vi "Get Data.vi"(8 "Error In":errorcluster, 11 "Model in":refnum<class "Model.lvclass">) -> (0 "Error Out":errorcluster, 2 "Digital Data":u8[](array[numeric]), 3 "Model out":refnum<class "Model.lvclass">)   [LabVIEW 2021, in "Model.lvclass"]
doc: "This VI enqueues a state to Analog to Digital Conversion VI which triggers it to send the U8 array data to Adc Viewer VI."
uses:
  Model.lvclass
  Controls/Queue Operation.ctl
  Controls/State Cluster.ctl
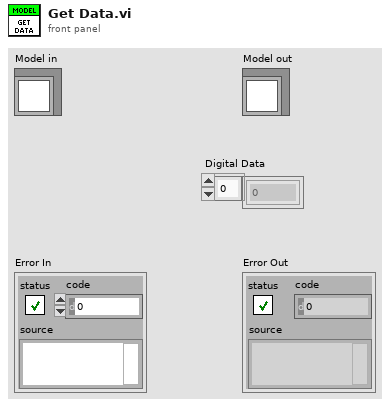
[diagram p1: front panel]
types:
  T1 = typedef "State Cluster.ctl" = cluster{"State":string, "Data":variant}
  T2 = typedef "Queue Operation.ctl" = enum16{"Create", "Enqueue", "Enqueue N", "Enstack", "Dequeue", "Flush", "Release"}
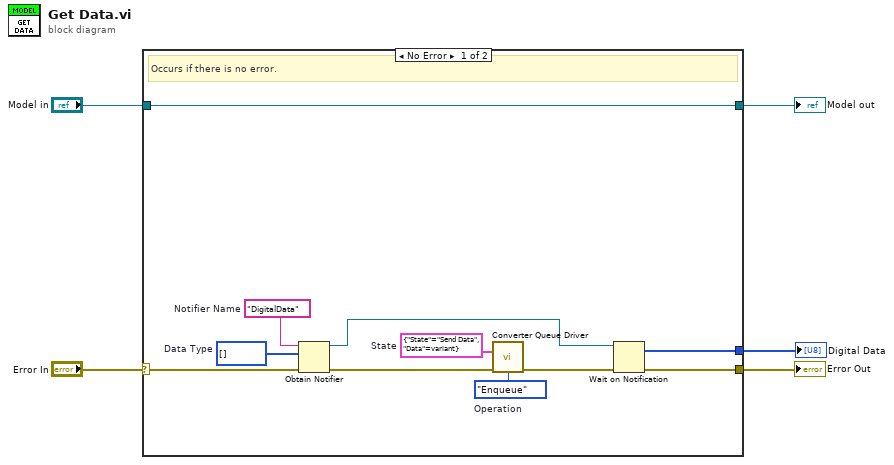
[diagram p0: block diagram]
diagram:
  n1 = case shown="No Error" "Error In" {
    selector: "Error In" -> [w11 w18]
    tunnel: [w8 w18] -> w4
    tunnel: [w16 w17] -> w2
    tunnel: "Model in" -> [w16 w17]
    tunnel: [w6 _] -> w1
    frame No Error {
      w9 = u8[] []  # Data Type
      w12 = "DigitalData"  # Notifier Name
      w14 = T1 {"State"="Send Data", "Data"=variant}  # State
      w15 = Queue_Operation."Enqueue"  # Operation
      # "Occurs if there is no error."
      n2 = Obtain Notifier(name (unnamed)=w12, notification data type=w9, error in (no error)=w11) -> (notifier out=w7:refnum<notifier>, error out=w10:errorcluster)  [unwired: 1 in, 1 out]
      n3 = call "Converter Queue Driver.vi"("State"=w14, "error in (no error)"=w10, "Operation"=w15) -> ("error out"=w13:errorcluster)  [unwired: 11 in, 1 out]
      n4 = Wait on Notification(notifier=w7, error in (no error)=w13) -> (notification=w6:u8[], error out=w8:errorcluster)  [unwired: 2 in, 2 out]
    }
    frame Error {
      # "Occurs if there is any error."
    }
  }
  "Error Out" <- w4
  "Model out" <- w2
  "Digital Data" <- w1
